vi "Read WT1600 VISA.vi"(8 "error in (no error)":errorcluster, 11 "WT1600 in":refnum<class "WT1600.lvclass">) -> (0 "error out":errorcluster, 2 "WT1600 VISA":refnum<visa-resource-name>, 3 "WT1600 out":refnum<class "WT1600.lvclass">)   [LabVIEW 2013, in "Universal Power Meter.lvlib" / "WT1600.lvlib" / "WT1600.lvclass"]
uses:
  WT1600.lvclass
  WT1600.lvclass/WT1600.ctl
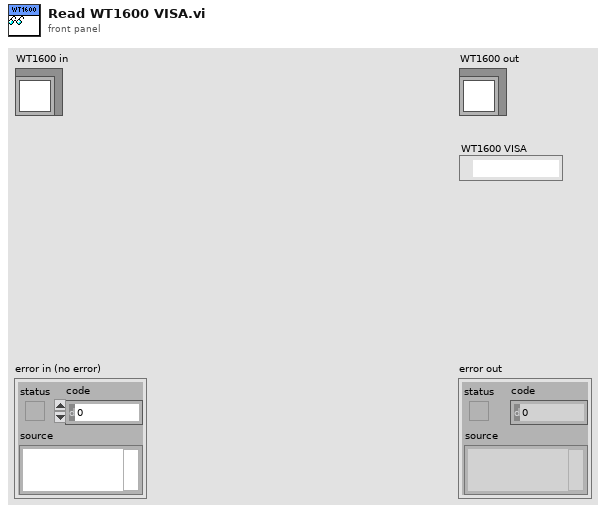
[diagram p1: front panel]
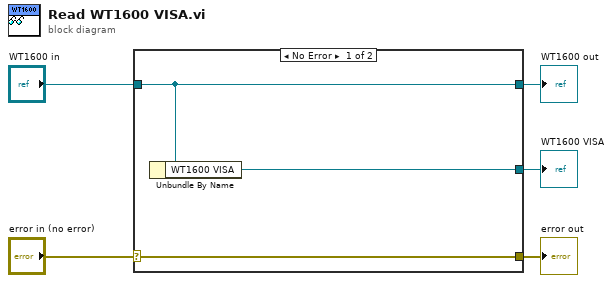
[diagram p0: block diagram]
diagram:
  n1 = case shown="No Error" "error in (no error)" {
    selector: "error in (no error)" -> [w8 w9]
    tunnel: [w8 w9] -> w4
    tunnel: [w7 w10] -> w2
    tunnel: "WT1600 in" -> [w7 w10]
    tunnel: [w6 _] -> w1
    frame No Error {
      n2 = Unbundle By Name(w7) -> ("WT1600 VISA"=w6:refnum<visa-resource-name>)
    }
    frame Error {
    }
  }
  "error out" <- w4
  "WT1600 out" <- w2
  "WT1600 VISA" <- w1
